vi "ILC Outputs View.vi"(10 "UserEvents in":refnum<class "UserEvents.lvclass">) -> ()   [LabVIEW 2015, in "FAMT Views.lvlib"]
uses:
  FAMT Views.lvlib
  <userlib>/Common/ILC/Typedefs/Outputs.ctl
  UserEvents/UserEvents.lvclass
  UserEvents/UserEvents.lvclass/UserEvents.ctl
  Typedefs/State Types.ctl
  Typedefs/FAMT Typedefs.lvlib
  <userlib>/Common/ILC/Typedefs/ILCTypedefs.lvlib
panel:
  out "ILC Outputs":T1 {"Step & Direction" min=-32767}
  # "DAC"
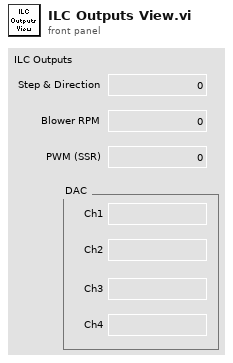
[diagram p1: front panel]
types:
  T1 = typedef "ILCCommon.lvlib/ILCTypedefs.lvlib/Outputs.ctl" = cluster{"Step & Direction":i16, "Blower RPM":u8, "PWM (SSR)":u8, "Ch1":u16, "Ch2":u16, "Ch3":u16, "Ch4":u16}
  T2 = typedef "FAMT Typedefs.lvlib/Publish Data Events.ctl" = cluster{"State":refnum<user-event>, "ErrorCode":refnum<user-event>, "FC1 ILC Outputs":refnum<user-event>, "LogPath":refnum<user-event>, "FC1 ILC Inputs":refnum<user-event>, "Scan Progress":refnum<user-event>, "FC2 ILC Outputs":refnum<user-event>, "FC2 ILC Inputs":refnum<user-event>}
  T3 = cluster{"Event Registration Refnum":refnum<event-registration>, "Event Registration Refnum":refnum<event-registration>}
  T4 = typedef "FAMT Typedefs.lvlib/State Types.ctl" = enum16{"Offline State", "Fault State", "Standby State", "Disabled State", "Enabled State", "Wait For User Input State", "Perform Open Loop Scan State", "Perform Closed Loop Scan State"}
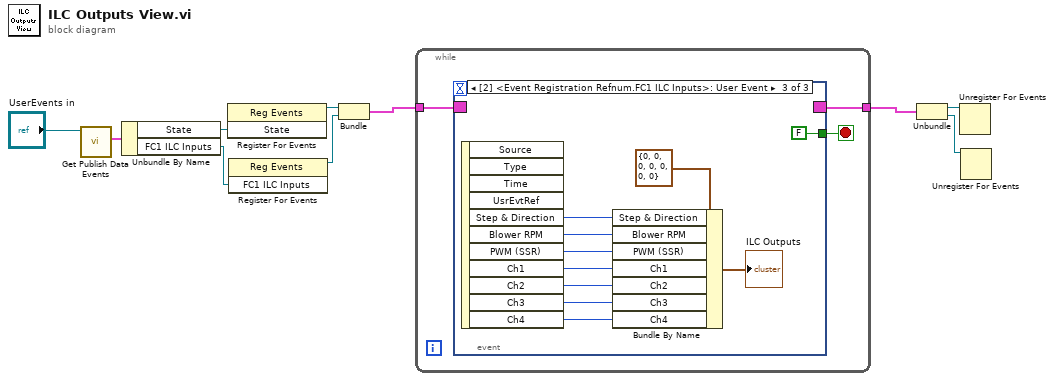
[diagram p0: block diagram]
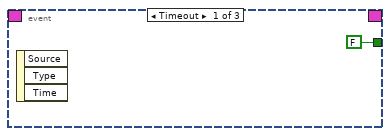
[diagram p2: hidden frame]
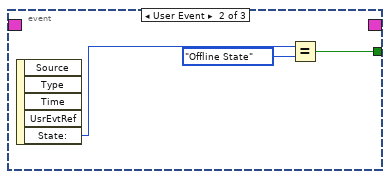
[diagram p3: hidden frame]
diagram:
  n1 = call "Get Publish Data Events.vi"("UserEvents in"="UserEvents in") -> ("Publish Data Events"=w4:T2)  [unwired: 9 in, 1 out]
  n2 = Unbundle By Name(w4) -> ("State"=w3:refnum<user-event>, "FC1 ILC Inputs"=w8:refnum<user-event>)
  n3 = register-events(w3) -> (reference out=w2:refnum<event-registration>)  [unwired: 2 in, 1 out]
  n4 = register-events(w8) -> (reference out=w9:refnum<event-registration>)  [unwired: 2 in, 1 out]
  n5 = Bundle("Event Registration Refnum"=w2, "Event Registration Refnum"=w9) -> (w5:T3)  [unwired: 1 in]
  n6 = while {
    tunnel: w5 -> [w13]
    tunnel: [w12] -> w7
    stop <- w11 stop-if-true
    n7 = event shown="[2] <Event Registration Refnum.FC1 ILC Inputs>: User Event" {
      selector: w13 -> [_ _ _]
      dyn-events: [_ _ _] -> w12
      timeout: _ -> [_ _ _]
      tunnel: [FALSE w15 FALSE] -> w11
      event Timeout {
        n8 = event-data() -> ()  [unwired: 1 in, 3 out]
      }
      event User Event {
        n9 = event-data() -> ("State:"=w17:T4)  [unwired: 1 in, 4 out]
        n10 = Equal?(x=w17, y=State_Types."Offline State") -> (x = y?=w15:bool)
      }
      event User Event {
        n11 = event-data() -> ("Step & Direction"=w20:i16, "Blower RPM"=w21:u8, "PWM (SSR)"=w22:u8, "Ch1"=w23:u16, "Ch2"=w24:u16, "Ch3"=w25:u16, "Ch4"=w26:u16)  [unwired: 1 in, 4 out]
        n12 = Bundle By Name(cluster=T1 {"Step & Direction"=0, "Blower RPM"=0, "PWM (SSR)"=0, "Ch1"=0, "Ch2"=0, "Ch3"=0, "Ch4"=0} ("ILC Outputs"), "Step & Direction"=w20, "Blower RPM"=w21, "PWM (SSR)"=w22, "Ch1"=w23, "Ch2"=w24, "Ch3"=w25, "Ch4"=w26) -> (→"ILC Outputs":T1)
      }
    }
  }
  n13 = Unbundle(w7) -> ("Event Registration Refnum"=w6:refnum<event-registration>, "Event Registration Refnum"=w10:refnum<event-registration>)
  n14 = Unregister For Events(event registration refnum=w6) -> ()  [unwired: 1 in, 1 out]
  n15 = Unregister For Events(event registration refnum=w10) -> ()  [unwired: 1 in, 1 out]
